vi "GetParent.vi"(8 "error in (no error)":errorcluster, 11 "Link in":refnum<class "Link.lvclass">) -> (0 "error out":errorcluster, 2 "parent GUID":string, 3 "Link out":refnum<class "Link.lvclass">)   [LabVIEW 2009, in "NavScreen.lvlib" / "Link.lvclass"]
uses:
  Link.lvclass
  Link.lvclass/Link.ctl
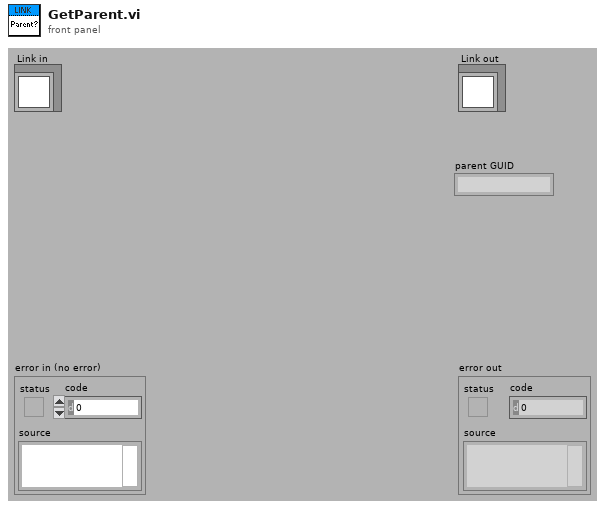
[diagram p1: front panel]
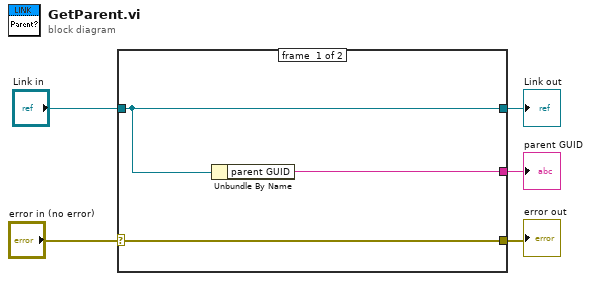
[diagram p0: block diagram]
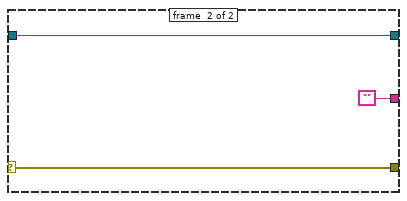
[diagram p2: hidden frame]
diagram:
  n1 = case shown="No Error" "error in (no error)" {
    selector: "error in (no error)" -> [w8 w11]
    tunnel: [w8 w11] -> w4
    tunnel: [w7 w10] -> w2
    tunnel: "Link in" -> [w7 w10]
    tunnel: [w6 "" ("Empty String Constant")] -> w1
    frame #0 {
      n2 = Unbundle By Name(w7) -> ("parent GUID"=w6:string)
    }
    frame #1 {
    }
  }
  "error out" <- w4
  "Link out" <- w2
  "parent GUID" <- w1
